vi "trio_read_limits.vi"(8 "error in (no error)":errorcluster, 10 "Axis":i32, 11 "Trio ref in":refnum<k7>) -> (0 "error out":errorcluster, 1 "Reverse Limit":bool, 2 "Forward Limit":bool, 3 "Trio ref out":refnum<k7>)   [LabVIEW 2017]
uses:
  <instrlib>/Trio Motion/Trio Motion Library.lvlib
panel:
  # "This will return an error out if at the limit"
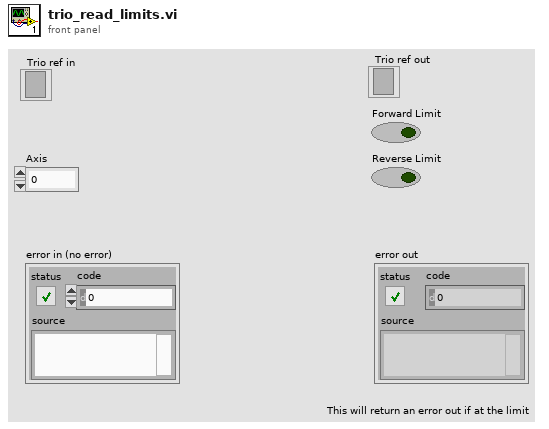
[diagram p1: front panel]
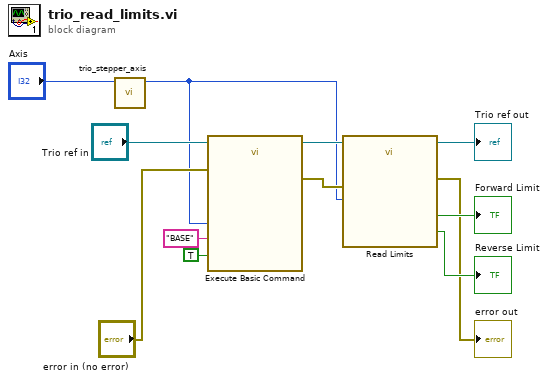
[diagram p0: block diagram]
diagram:
  n1 = call "trio_stepper_axis.vi"("Encoder axis"="Axis") -> ("Stepper axis"=w2:i32)  [unwired: 10 in]
  n2 = call <instrlib>:"Execute Basic Command.vi"("Include Value (F)"=TRUE, "error in (no error)"="error in (no error)", "Value"=w2, "Command"="BASE", "reference in"="Trio ref in") -> ("error out"=w9:errorcluster, "reference out"=w10:refnum<k7>)  [unwired: 4 in, 1 out]
  n3 = call <instrlib>:"Read Limits.vi"("reference in"=w10, "Axis (0)"=w2, "error in (no error)"=w9) -> ("reference out"=→"Trio ref out":refnum<k7>, "Forward Limit"=→"Forward Limit":bool, "Reverse Limit"=→"Reverse Limit":bool, "error out"=→"error out":errorcluster)  [unwired: 7 in, 2 out]
